vi "PH_StatusHandler.calc Status out of endswitches.vi"(2 "Status Input 2: \"True\"":T1 caption="Input 2" items=["no info", "off/false/out", "on/true/in", "Failure", "Alarm", "Status 1", "Status 2", "Status 3"], 3 "Status Input 1: \"False\"":T1 caption="Input 1" items=["no info", "off/false/out", "on/true/in", "Failure", "Alarm", "Status 1", "Status 2", "Status 3"]) -> (0 "Further Information":string, 1 "Status Output":T1 caption="Result" items=["no info", "off/false/out", "on/true/in", "Failure", "Alarm", "Status 1", "Status 2", "Status 3"])   [LabVIEW 2014, in "PH_StatusHandler.lvlib"]
doc: "This VI calculates the resultung status of a switch with two - a false and a true \"endswitch\" inputs:\n\nIf one input is alarm, the output is alarm (Further information: \"at least one alarm\").\nIf one input is failure, the outout is failure (\"at least one failure\").\nIf \"false\" input is true and the other false, the output is off/false/out (\"false\").\nIf \"false\" input is false and the other true, the output is on/true/in (\"true\").\nIf both inputs are false, the output is Status 1 (\"in between\").\nIf both inputs are true, the output is Failure (\"Failure\").\nElse: output is no info (\"no info\")."
uses:
  PH_StatusHandler.Status.ctl
  PH_StatusHandler.lvlib
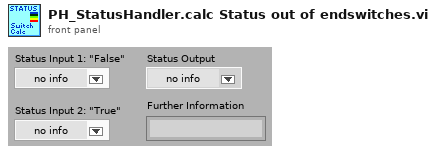
[diagram p1: front panel]
types:
  T1 = typedef "PH_StatusHandler.lvlib/PH_StatusHandler.Status.ctl" = i16
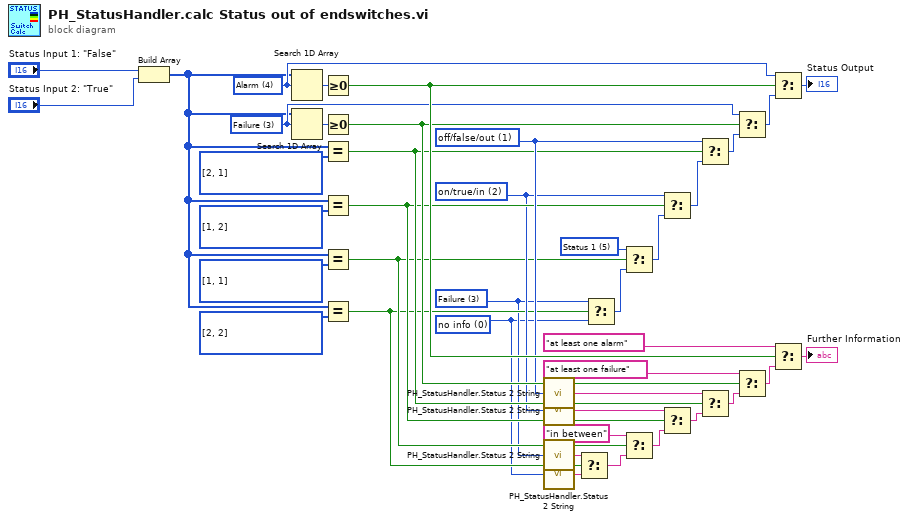
[diagram p0: block diagram]
diagram:
  w4 = T1 3 items=["no info", "off/false/out", "on/true/in", "Failure", "Alarm", "Status 1", "Status 2", "Status 3"] ("Status Input 2: \"True\"")
  w9 = T1[] [2, 2] items=["no info", "off/false/out", "on/true/in", "Failure", "Alarm", "Status 1", "Status 2", "Status 3"] ("y")
  w13 = T1 5 items=["no info", "off/false/out", "on/true/in", "Failure", "Alarm", "Status 1", "Status 2", "Status 3"] ("Status Input 2: \"True\"")
  w15 = T1[] [1, 1] items=["no info", "off/false/out", "on/true/in", "Failure", "Alarm", "Status 1", "Status 2", "Status 3"] ("y")
  w16 = T1 2 items=["no info", "off/false/out", "on/true/in", "Failure", "Alarm", "Status 1", "Status 2", "Status 3"] ("Status Input 2: \"True\"")
  w21 = T1[] [1, 2] items=["no info", "off/false/out", "on/true/in", "Failure", "Alarm", "Status 1", "Status 2", "Status 3"] ("y")
  w24 = T1 1 items=["no info", "off/false/out", "on/true/in", "Failure", "Alarm", "Status 1", "Status 2", "Status 3"] ("Status Input 2: \"True\"")
  w27 = T1[] [2, 1] items=["no info", "off/false/out", "on/true/in", "Failure", "Alarm", "Status 1", "Status 2", "Status 3"] ("y")
  w2 = T1 0 items=["no info", "off/false/out", "on/true/in", "Failure", "Alarm", "Status 1", "Status 2", "Status 3"] ("Status Input 2: \"True\"")
  w32 = T1 3 items=["no info", "off/false/out", "on/true/in", "Failure", "Alarm", "Status 1", "Status 2", "Status 3"] ("Status Input 2: \"True\"")
  w34 = T1 4 items=["no info", "off/false/out", "on/true/in", "Failure", "Alarm", "Status 1", "Status 2", "Status 3"] ("Status Input 2: \"True\"")
  n1 = Build Array("Status Input 1: \"False\"", "Status Input 2: \"True\"") -> (w8:T1[])
  n2 = Search 1D Array(1D array=w8, element=w34) -> (index of element=w39:i32)  [unwired: 1 in]
  n3 = Search 1D Array(1D array=w8, element=w32) -> (index of element=w33:i32)  [unwired: 1 in]
  n4 = Greater Or Equal To 0?(x=w39) -> (x >= 0?=w37:bool)
  n5 = Greater Or Equal To 0?(x=w33) -> (x >= 0?=w29:bool)
  n6 = Equal?(x=w8, y=w27) -> (x = y?=w22:bool)
  n7 = Equal?(x=w8, y=w21) -> (x = y?=w18:bool)
  n8 = Equal?(x=w8, y=w15) -> (x = y?=w12:bool)
  n9 = Equal?(x=w8, y=w9) -> (x = y?=w5:bool)
  n10 = call "PH_StatusHandler.Status 2 String.vi"("Status"=w24) -> ("Status as string"=w23:string)
  n11 = call "PH_StatusHandler.Status 2 String.vi"("Status"=w16) -> ("Status as string"=w17:string)
  n12 = call "PH_StatusHandler.Status 2 String.vi"("Status"=w4) -> ("Status as string"=w3:string)
  n13 = call "PH_StatusHandler.Status 2 String.vi"("Status"=w2) -> ("Status as string"=w1:string)
  n14 = Select(t=w3, s=w5, f=w1) -> (s? t:f=w6:string)
  n15 = Select(t=w4, s=w5, f=w2) -> (s? t:f=w7:T1)
  n16 = Select(t=w13, s=w12, f=w7) -> (s? t:f=w14:T1)
  n17 = Select(t="in between", s=w12, f=w6) -> (s? t:f=w11:string)
  n18 = Select(t=w16, s=w18, f=w14) -> (s? t:f=w20:T1)
  n19 = Select(t=w17, s=w18, f=w11) -> (s? t:f=w19:string)
  n20 = Select(t=w24, s=w22, f=w20) -> (s? t:f=w26:T1)
  n21 = Select(t=w23, s=w22, f=w19) -> (s? t:f=w25:string)
  n22 = Select(t=w32, s=w29, f=w26) -> (s? t:f=w31:T1)
  n23 = Select(t="at least one failure", s=w29, f=w25) -> (s? t:f=w30:string)
  n24 = Select(t=w34, s=w37, f=w31) -> (s? t:f=→"Status Output":T1)
  n25 = Select(t="at least one alarm", s=w37, f=w30) -> (s? t:f=→"Further Information":string)
